vi "基础13.vi"() -> ()   [LabVIEW 2014]
panel:
  in  "停止":bool
  out "布尔":bool
  in  "数值":dbl
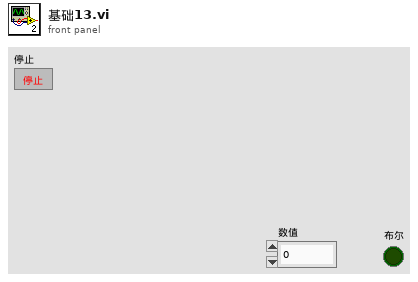
[diagram p1: front panel]
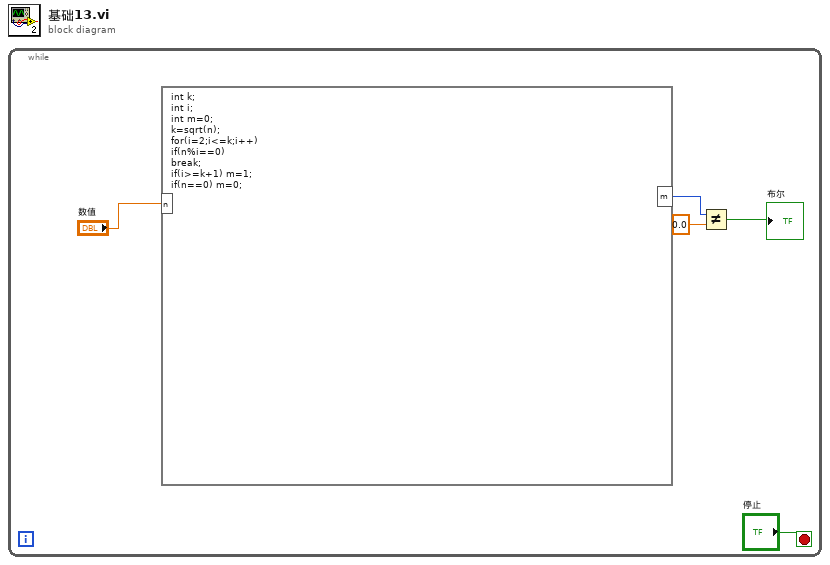
[diagram p0: block diagram]
diagram:
  n1 = while {
    stop <- "停止" stop-if-true
    n2 = formula code="int k;\nint i;\nint m=0;\nk=sqrt(n);\nfor(i=2;i<=k;i++) \nif(n%i==0) \nbreak;\nif(i>=k+1) m=1;\nif(n==0) m=0;"("n"="数值") -> ("m"=w3:i32)
    n3 = Not Equal?(x=w3, y=0.0) -> (x != y?=→"布尔":bool)
  }
